vi "Measurement Logic.vi"() -> ()   [LabVIEW 2024, in "NIScopeTimeDomain.lvlib"]
uses:
  NIScopeTimeDomain.lvlib
  <vilib>/MeasurementLink/MeasurementLink Measurement Server/Measure Call Context/Measure Call Context.lvclass
  <vilib>/MeasurementLink/MeasurementLink niScope/MeasurementLink niScope.lvlib
  <vilib>/MeasurementLink/MeasurementLink Session Management V1/Session Reservation/Session Reservation.lvclass
  Measurement Results.ctl
  <instrlib>/niScope/Measurements/niScope Fetch Measurement Stats.vi
  <instrlib>/niScope/Controls/niScope scalar measurement.ctl
  <instrlib>/niScope/Acquire/Fetch/niScope Fetch WDT.vi
  <instrlib>/niScope/Configure/Trigger/niScope Configure Trigger Edge.vi
  <vilib>/MeasurementLink/MeasurementLink niScope/Get Connections - 1Pin 1Conn.vi
  <vilib>/MeasurementLink/MeasurementLink niScope/Initialize Sessions - 1Sess.vi
  <vilib>/MeasurementLink/MeasurementLink Measurement Server/Measure Call Context/Reserve Sessions - 1Pin.vi
  Measurement Configuration.ctl
panel:
  out "measurement results":T1
  out "measure call context out":refnum<class "Measure Call Context.lvclass">
  in  "measure call context in":refnum<class "Measure Call Context.lvclass">
  in  "measurement configuration":T2={"Pin Name"="", "Vertical Range (V)"=10.0, "Vertical Offset (V)"=0.0, "Vertical Coupling"=1, "Minimum Sample Rate (S/s)"=10000.0, "Minimum Record Length (S)"=20000, "Trigger Level (V)"=0.5, "Trigger Coupling"=0, "Trigger Slope"=1} {"Trigger Slope" items=["AC"=0, "DC"=1, "HF Reject"=3, "LF Reject"=4, "AC Plus HF Reject"=1001]; "Trigger Coupling" items=["Positive", "Negative"]; "Vertical Coupling" items=["AC", "DC", "Ground"]; "Vertical Offset (V)" format="%.2p"}
  out "error out":errorcluster
  in  "error in":errorcluster
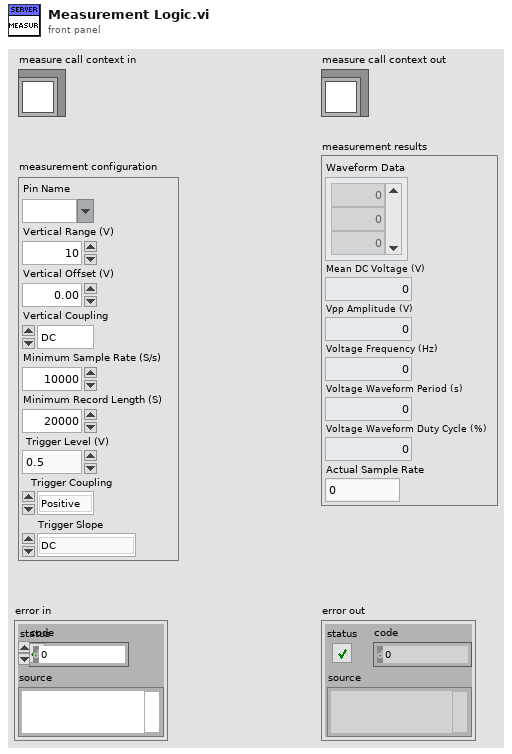
[diagram p1: front panel]
types:
  T1 = typedef "NIScopeTimeDomain.lvlib/Measurement Results.ctl" = cluster{"Waveform Data":dbl[], "Mean DC Voltage (V)":dbl, "Vpp Amplitude (V)":dbl, "Voltage Frequency (Hz)":dbl, "Voltage Waveform Period (s)":dbl, "Voltage Waveform Duty Cycle (%)":dbl, "Actual Sample Rate":dbl}
  T2 = typedef "NIScopeTimeDomain.lvlib/Measurement Configuration.ctl" = cluster{"Pin Name":string, "Vertical Range (V)":dbl, "Vertical Offset (V)":dbl, "Vertical Coupling":i32, "Minimum Sample Rate (S/s)":dbl, "Minimum Record Length (S)":i32, "Trigger Level (V)":dbl, "Trigger Coupling":u32, "Trigger Slope":i32}
  T3 = typedef "niScope scalar measurement.ctl" = i32
  T4 = typedef "MeasurementLink niScope.lvlib/Connection with Session.ctl" = cluster{"connection":T5, "session":refnum<k15>}
  T5 = typedef "MeasurementLink Session Management V1.lvlib/Session Reservation.lvclass/Connection.ctl" = cluster{"pin or relay name":string, "site":i32, "instrument type id":string, "channel":string}
  T6 = cluster{"result":dbl, "mean":dbl, "stdev":dbl, "min":dbl, "max":dbl, "num in stats":i32}
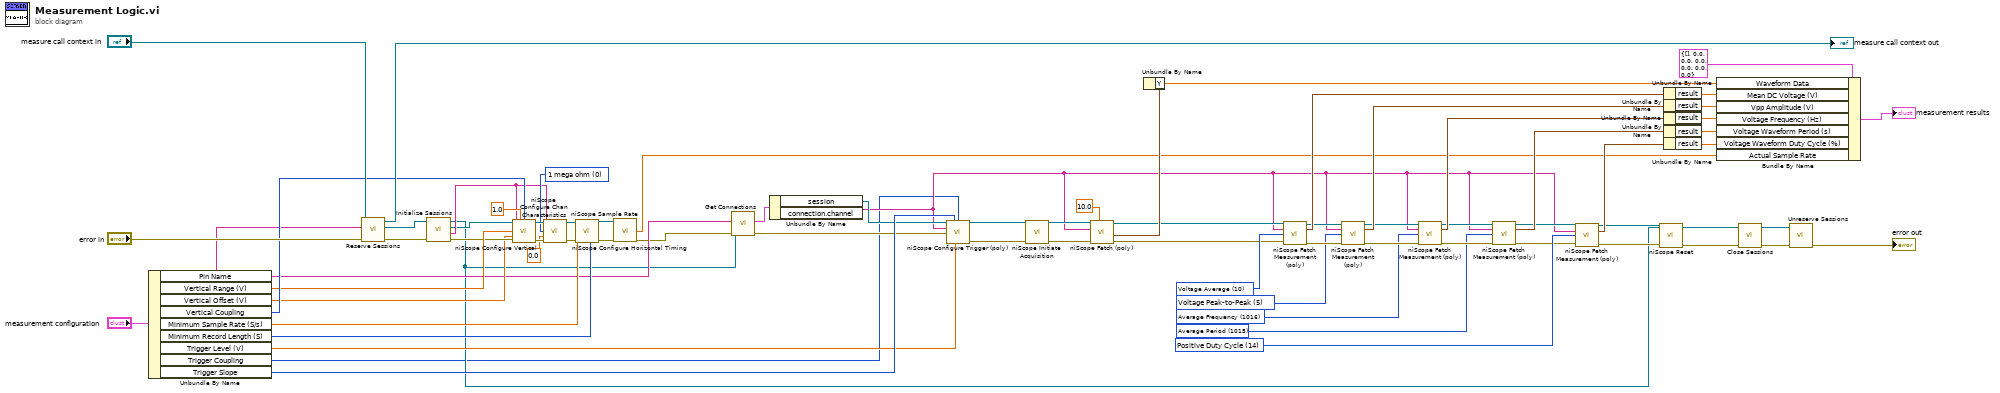
[diagram p0: block diagram]
diagram:
  w12 = T3 1015 items=["None"=4000, "Frequency"=2, "Average Frequency"=1016, "FFT Frequency"=1008, "Period"=3, "Average Period"=1015, "Rise Time"=0, "Fall Time"=1, "Rising Slew Rate"=1010, "Falling Slew Rate"=1011, "Overshoot"=18, "Preshoot"=19, "Voltage RMS"=4, "Voltage Cycle RMS"=16, "AC Estimate"=1012, "FFT Amplitude"=1009, "Voltage Average"=10, "Voltage Cycle Average"=17, "DC Estimate"=1013, "Voltage Max"=6, "Voltage Min"=7, "Voltage Peak-to-Peak"=5, "Voltage High"=8, "Voltage Low"=9, "Voltage Amplitude"=15, "Voltage Top"=1007, "Voltage Base"=1006, "Voltage Base-to-Top"=1017, "Negative Width"=11, "Positive Width"=12, "Negative Duty Cycle"=13, "Positive Duty Cycle"=14, "Integral"=1005, "Area"=1003, "Cycle Area"=1004, "Time Delay"=1014, "Phase Delay"=1018, "Low Ref Volts"=1000, "Mid Ref Volts"=1001, "High Ref Volts"=1002, "Volt. Hist. Mean"=2000, "Volt. Hist. Stdev"=2001, "Volt. Hist. Median"=2003, "Volt. Hist. Mode"=2010, "Volt. Hist. Max"=2005, "Volt. Hist. Min"=2006, "Volt. Hist. Peak-to-Peak"=2002, "Volt. Hist. Mean + Stdev"=2007, "Volt. Hist. Mean + 2 Stdev"=2008, "Volt. Hist. Mean + 3 Stdev"=2009, "Volt. Hist. Hits"=2004, "Volt. Hist. New Hits"=2011, "Time Hist. Mean"=3000, "Time Hist. Stdev"=3001, "Time Hist. Median"=3003, "Time Hist. Mode"=3010, "Time Hist. Max"=3005, "Time Hist. Min"=3006, "Time Hist. Peak-to-Peak"=3002, "Time Hist. Mean + Stdev"=3007, "Time Hist. Mean + 2 Stdev"=3008, "Time Hist. Mean + 3 Stdev"=3009, "Time Hist. Hits"=3004, "Time Hist. New Hits"=3011] ("scalar measurement")
  w23 = T3 14 items=["None"=4000, "Frequency"=2, "Average Frequency"=1016, "FFT Frequency"=1008, "Period"=3, "Average Period"=1015, "Rise Time"=0, "Fall Time"=1, "Rising Slew Rate"=1010, "Falling Slew Rate"=1011, "Overshoot"=18, "Preshoot"=19, "Voltage RMS"=4, "Voltage Cycle RMS"=16, "AC Estimate"=1012, "FFT Amplitude"=1009, "Voltage Average"=10, "Voltage Cycle Average"=17, "DC Estimate"=1013, "Voltage Max"=6, "Voltage Min"=7, "Voltage Peak-to-Peak"=5, "Voltage High"=8, "Voltage Low"=9, "Voltage Amplitude"=15, "Voltage Top"=1007, "Voltage Base"=1006, "Voltage Base-to-Top"=1017, "Negative Width"=11, "Positive Width"=12, "Negative Duty Cycle"=13, "Positive Duty Cycle"=14, "Integral"=1005, "Area"=1003, "Cycle Area"=1004, "Time Delay"=1014, "Phase Delay"=1018, "Low Ref Volts"=1000, "Mid Ref Volts"=1001, "High Ref Volts"=1002, "Volt. Hist. Mean"=2000, "Volt. Hist. Stdev"=2001, "Volt. Hist. Median"=2003, "Volt. Hist. Mode"=2010, "Volt. Hist. Max"=2005, "Volt. Hist. Min"=2006, "Volt. Hist. Peak-to-Peak"=2002, "Volt. Hist. Mean + Stdev"=2007, "Volt. Hist. Mean + 2 Stdev"=2008, "Volt. Hist. Mean + 3 Stdev"=2009, "Volt. Hist. Hits"=2004, "Volt. Hist. New Hits"=2011, "Time Hist. Mean"=3000, "Time Hist. Stdev"=3001, "Time Hist. Median"=3003, "Time Hist. Mode"=3010, "Time Hist. Max"=3005, "Time Hist. Min"=3006, "Time Hist. Peak-to-Peak"=3002, "Time Hist. Mean + Stdev"=3007, "Time Hist. Mean + 2 Stdev"=3008, "Time Hist. Mean + 3 Stdev"=3009, "Time Hist. Hits"=3004, "Time Hist. New Hits"=3011] ("scalar measurement")
  w24 = T3 1016 items=["None"=4000, "Frequency"=2, "Average Frequency"=1016, "FFT Frequency"=1008, "Period"=3, "Average Period"=1015, "Rise Time"=0, "Fall Time"=1, "Rising Slew Rate"=1010, "Falling Slew Rate"=1011, "Overshoot"=18, "Preshoot"=19, "Voltage RMS"=4, "Voltage Cycle RMS"=16, "AC Estimate"=1012, "FFT Amplitude"=1009, "Voltage Average"=10, "Voltage Cycle Average"=17, "DC Estimate"=1013, "Voltage Max"=6, "Voltage Min"=7, "Voltage Peak-to-Peak"=5, "Voltage High"=8, "Voltage Low"=9, "Voltage Amplitude"=15, "Voltage Top"=1007, "Voltage Base"=1006, "Voltage Base-to-Top"=1017, "Negative Width"=11, "Positive Width"=12, "Negative Duty Cycle"=13, "Positive Duty Cycle"=14, "Integral"=1005, "Area"=1003, "Cycle Area"=1004, "Time Delay"=1014, "Phase Delay"=1018, "Low Ref Volts"=1000, "Mid Ref Volts"=1001, "High Ref Volts"=1002, "Volt. Hist. Mean"=2000, "Volt. Hist. Stdev"=2001, "Volt. Hist. Median"=2003, "Volt. Hist. Mode"=2010, "Volt. Hist. Max"=2005, "Volt. Hist. Min"=2006, "Volt. Hist. Peak-to-Peak"=2002, "Volt. Hist. Mean + Stdev"=2007, "Volt. Hist. Mean + 2 Stdev"=2008, "Volt. Hist. Mean + 3 Stdev"=2009, "Volt. Hist. Hits"=2004, "Volt. Hist. New Hits"=2011, "Time Hist. Mean"=3000, "Time Hist. Stdev"=3001, "Time Hist. Median"=3003, "Time Hist. Mode"=3010, "Time Hist. Max"=3005, "Time Hist. Min"=3006, "Time Hist. Peak-to-Peak"=3002, "Time Hist. Mean + Stdev"=3007, "Time Hist. Mean + 2 Stdev"=3008, "Time Hist. Mean + 3 Stdev"=3009, "Time Hist. Hits"=3004, "Time Hist. New Hits"=3011] ("scalar measurement")
  w27 = T3 5 items=["None"=4000, "Frequency"=2, "Average Frequency"=1016, "FFT Frequency"=1008, "Period"=3, "Average Period"=1015, "Rise Time"=0, "Fall Time"=1, "Rising Slew Rate"=1010, "Falling Slew Rate"=1011, "Overshoot"=18, "Preshoot"=19, "Voltage RMS"=4, "Voltage Cycle RMS"=16, "AC Estimate"=1012, "FFT Amplitude"=1009, "Voltage Average"=10, "Voltage Cycle Average"=17, "DC Estimate"=1013, "Voltage Max"=6, "Voltage Min"=7, "Voltage Peak-to-Peak"=5, "Voltage High"=8, "Voltage Low"=9, "Voltage Amplitude"=15, "Voltage Top"=1007, "Voltage Base"=1006, "Voltage Base-to-Top"=1017, "Negative Width"=11, "Positive Width"=12, "Negative Duty Cycle"=13, "Positive Duty Cycle"=14, "Integral"=1005, "Area"=1003, "Cycle Area"=1004, "Time Delay"=1014, "Phase Delay"=1018, "Low Ref Volts"=1000, "Mid Ref Volts"=1001, "High Ref Volts"=1002, "Volt. Hist. Mean"=2000, "Volt. Hist. Stdev"=2001, "Volt. Hist. Median"=2003, "Volt. Hist. Mode"=2010, "Volt. Hist. Max"=2005, "Volt. Hist. Min"=2006, "Volt. Hist. Peak-to-Peak"=2002, "Volt. Hist. Mean + Stdev"=2007, "Volt. Hist. Mean + 2 Stdev"=2008, "Volt. Hist. Mean + 3 Stdev"=2009, "Volt. Hist. Hits"=2004, "Volt. Hist. New Hits"=2011, "Time Hist. Mean"=3000, "Time Hist. Stdev"=3001, "Time Hist. Median"=3003, "Time Hist. Mode"=3010, "Time Hist. Max"=3005, "Time Hist. Min"=3006, "Time Hist. Peak-to-Peak"=3002, "Time Hist. Mean + Stdev"=3007, "Time Hist. Mean + 2 Stdev"=3008, "Time Hist. Mean + 3 Stdev"=3009, "Time Hist. Hits"=3004, "Time Hist. New Hits"=3011] ("scalar measurement")
  w35 = T3 10 items=["None"=4000, "Frequency"=2, "Average Frequency"=1016, "FFT Frequency"=1008, "Period"=3, "Average Period"=1015, "Rise Time"=0, "Fall Time"=1, "Rising Slew Rate"=1010, "Falling Slew Rate"=1011, "Overshoot"=18, "Preshoot"=19, "Voltage RMS"=4, "Voltage Cycle RMS"=16, "AC Estimate"=1012, "FFT Amplitude"=1009, "Voltage Average"=10, "Voltage Cycle Average"=17, "DC Estimate"=1013, "Voltage Max"=6, "Voltage Min"=7, "Voltage Peak-to-Peak"=5, "Voltage High"=8, "Voltage Low"=9, "Voltage Amplitude"=15, "Voltage Top"=1007, "Voltage Base"=1006, "Voltage Base-to-Top"=1017, "Negative Width"=11, "Positive Width"=12, "Negative Duty Cycle"=13, "Positive Duty Cycle"=14, "Integral"=1005, "Area"=1003, "Cycle Area"=1004, "Time Delay"=1014, "Phase Delay"=1018, "Low Ref Volts"=1000, "Mid Ref Volts"=1001, "High Ref Volts"=1002, "Volt. Hist. Mean"=2000, "Volt. Hist. Stdev"=2001, "Volt. Hist. Median"=2003, "Volt. Hist. Mode"=2010, "Volt. Hist. Max"=2005, "Volt. Hist. Min"=2006, "Volt. Hist. Peak-to-Peak"=2002, "Volt. Hist. Mean + Stdev"=2007, "Volt. Hist. Mean + 2 Stdev"=2008, "Volt. Hist. Mean + 3 Stdev"=2009, "Volt. Hist. Hits"=2004, "Volt. Hist. New Hits"=2011, "Time Hist. Mean"=3000, "Time Hist. Stdev"=3001, "Time Hist. Median"=3003, "Time Hist. Mode"=3010, "Time Hist. Max"=3005, "Time Hist. Min"=3006, "Time Hist. Peak-to-Peak"=3002, "Time Hist. Mean + Stdev"=3007, "Time Hist. Mean + 2 Stdev"=3008, "Time Hist. Mean + 3 Stdev"=3009, "Time Hist. Hits"=3004, "Time Hist. New Hits"=3011] ("scalar measurement")
  w58 = u32 0 items=["1 mega ohm"=0, "50 ohms"=2] ("input impedance")
  n1 = Unbundle By Name("measurement configuration") -> ("Pin Name"=w39:string, "Vertical Range (V)"=w64:dbl, "Vertical Offset (V)"=w62:dbl, "Vertical Coupling"=w68:i32, "Minimum Sample Rate (S/s)"=w55:dbl, "Minimum Record Length (S)"=w53:i32, "Trigger Level (V)"=w51:dbl, "Trigger Coupling"=w5:u32, "Trigger Slope"=w52:i32)
  n2 = call-poly <vilib>:"Reserve Sessions.vi"("error in"="error in", "pin or relay name"=w39, "measurement context in"="measure call context in") -> ("error out"=w70:errorcluster, "session reservation out"=w71:refnum<class "Session Reservation.lvclass">, "measurement context out"=→"measure call context out":refnum<class "Measure Call Context.lvclass">)  [unwired: 6 in]
  n3 = call-poly <vilib>:"Initialize Sessions.vi"("error in"=w70, "session reservation in"=w71) -> ("error out"=w63:errorcluster, "channel list"=w56:string, "session"=w49:refnum<k15>, "session reservation out"=w6:refnum<class "Session Reservation.lvclass">)  [unwired: 6 in]
  n4 = call <instrlib>:"niScope Configure Vertical.vi"("instrument handle"=w49, "probe attenuation"=1.0, "vertical coupling"=w68, "channels"=w56, "vertical range"=w64, "vertical offset"=w62, "error in"=w63) -> ("instrument handle out"=w60:refnum<k15>, "error out"=w59:errorcluster)  [unwired: 7 in]
  n5 = call <instrlib>:"niScope Configure Chan Characteristics.vi"("instrument handle"=w60, "channels"=w56, "input impedance"=w58, "maximum input frequency"=0.0, "error in"=w59) -> ("instrument handle out"=w44:refnum<k15>, "error out"=w54:errorcluster)  [unwired: 9 in]
  n6 = call <instrlib>:"niScope Configure Horizontal Timing.vi"("instrument handle"=w44, "min sample rate"=w55, "error in"=w54, "min record length"=w53) -> ("instrument handle out"=w2:refnum<k15>, "error out"=w4:errorcluster)  [unwired: 10 in]
  n7 = call <instrlib>:"niScope Sample Rate.vi"("instrument handle"=w2, "error in"=w4) -> ("actual sample rate"=w1:dbl, "error out"=w3:errorcluster)  [unwired: 11 in, 1 out]
  n8 = call-poly <vilib>:"Get Connections.vi"("error in"=w3, "pin or relay name"=w39, "session reservation in"=w6) -> ("error out"=w38:errorcluster, "connection"=w37:T4)  [unwired: 6 in, 1 out]
  n9 = Unbundle By Name(w37) -> ("session"=w36:refnum<k15>, "connection.channel"=w7:string)
  n10 = call-poly <instrlib>:"niScope Configure Trigger (poly).vi"("instrument handle"=w36, "trigger slope"=w52, "trigger coupling"=w5, "trigger source"=w7, "trigger level"=w51, "error in"=w38) -> ("instrument handle out"=w48:refnum<k15>, "error out"=w50:errorcluster)  [unwired: 8 in]
  n11 = call <instrlib>:"niScope Initiate Acquisition.vi"("instrument handle"=w48, "error in"=w50) -> ("instrument handle out"=w47:refnum<k15>, "error out"=w46:errorcluster)  [unwired: 12 in]
  n12 = call-poly <instrlib>:"niScope Fetch (poly).vi"("timeout"=10.0, "error in"=w46, "channels"=w7, "instrument handle"=w47) -> ("error out"=w32:errorcluster, "wfm"=w43:waveform(dbl), "instrument handle out"=w11:refnum<k15>)  [unwired: 4 in, 1 out]
  n13 = Unbundle By Name(w43) -> ("Y"=w42:dbl[])
  n14 = call-poly <instrlib>:"niScope Fetch Measurement (poly).vi"("instrument handle"=w11, "channels"=w7, "scalar measurement"=w35, "error in"=w32) -> ("instrument handle out"=w31:refnum<k15>, "stats"=w34:T6, "error out"=w28:errorcluster)  [unwired: 9 in]
  n15 = call-poly <instrlib>:"niScope Fetch Measurement (poly).vi"("instrument handle"=w31, "channels"=w7, "scalar measurement"=w27, "error in"=w28) -> ("instrument handle out"=w26:refnum<k15>, "stats"=w30:T6, "error out"=w25:errorcluster)  [unwired: 9 in]
  n16 = call-poly <instrlib>:"niScope Fetch Measurement (poly).vi"("instrument handle"=w26, "channels"=w7, "scalar measurement"=w24, "error in"=w25) -> ("instrument handle out"=w13:refnum<k15>, "stats"=w22:T6, "error out"=w17:errorcluster)  [unwired: 9 in]
  n17 = call-poly <instrlib>:"niScope Fetch Measurement (poly).vi"("instrument handle"=w13, "channels"=w7, "scalar measurement"=w12, "error in"=w17) -> ("instrument handle out"=w14:refnum<k15>, "stats"=w15:T6, "error out"=w18:errorcluster)  [unwired: 9 in]
  n18 = call-poly <instrlib>:"niScope Fetch Measurement (poly).vi"("instrument handle"=w14, "channels"=w7, "scalar measurement"=w23, "error in"=w18) -> ("instrument handle out"=w9:refnum<k15>, "stats"=w19:T6, "error out"=w8:errorcluster)  [unwired: 9 in]
  n19 = call <instrlib>:"niScope Reset.vi"("instrument handle"=w9, "error in"=w8) -> ("error out"=w10:errorcluster)  [unwired: 12 in, 1 out]
  n20 = Unbundle By Name(w34) -> ("result"=w33:dbl)
  n21 = Unbundle By Name(w30) -> ("result"=w29:dbl)
  n22 = Unbundle By Name(w22) -> ("result"=w21:dbl)
  n23 = Unbundle By Name(w15) -> ("result"=w16:dbl)
  n24 = Unbundle By Name(w19) -> ("result"=w20:dbl)
  n25 = Bundle By Name(cluster=T1 {"Waveform Data"=[], "Mean DC Voltage (V)"=0.0, "Vpp Amplitude (V)"=0.0, "Voltage Frequency (Hz)"=0.0, "Voltage Waveform Period (s)"=0.0, "Voltage Waveform Duty Cycle (%)"=0.0, "Actual Sample Rate"=0.0} ("measurement results"), "Waveform Data"=w42, "Mean DC Voltage (V)"=w33, "Vpp Amplitude (V)"=w29, "Voltage Frequency (Hz)"=w21, "Voltage Waveform Period (s)"=w16, "Voltage Waveform Duty Cycle (%)"=w20, "Actual Sample Rate"=w1) -> (→"measurement results":T1)
  n26 = call <vilib>:"Close Sessions.vi"("error in"=w10, "session reservation in"=w6) -> ("error out"=w65:errorcluster, "session reservation out"=w67:refnum<class "Session Reservation.lvclass">)  [unwired: 8 in]
  n27 = call <vilib>:"Unreserve Sessions.vi"("error in"=w65, "session reservation in"=w67) -> ("error out"=→"error out":errorcluster)  [unwired: 9 in]
